vi "Write Topic Filter.vi"(8 "error in (no error)":errorcluster, 10 "Topic Filter":string, 11 "Subscription in":refnum<class "Subscription.lvclass">) -> (0 "error out":errorcluster, 3 "Subscription out":refnum<class "Subscription.lvclass">)   [LabVIEW 2013, in "MQTT Server.lvlib" / "Subscription.lvclass"]
uses:
  Subscription.lvclass
  Subscription.lvclass/Subscription.ctl
  TopicFilter/TopicFilter.lvclass/TopicFilter.ctl
  TopicFilter/TopicFilter.lvclass
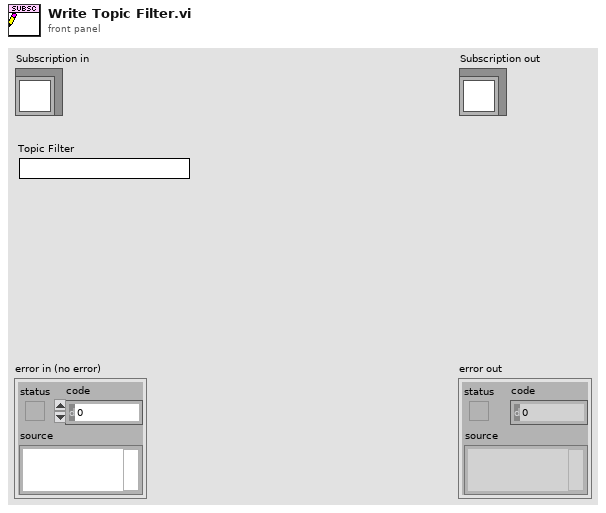
[diagram p1: front panel]
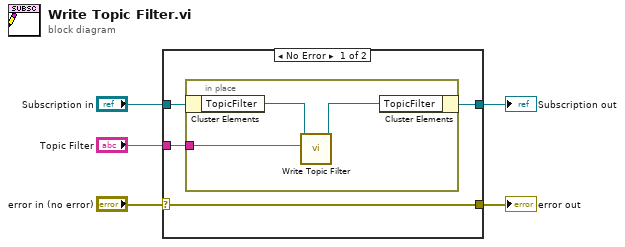
[diagram p0: block diagram]
diagram:
  n1 = case shown="No Error" "error in (no error)" {
    selector: "error in (no error)" -> [w9 w13]
    tunnel: [w9 w13] -> w4
    tunnel: [w6 w14] -> w2
    tunnel: "Subscription in" -> [w7 w14]
    tunnel: "Topic Filter" -> [w8 _]
    frame No Error {
      n2 = in-place {
        in-place-border: w8 -> [w12]
        n3 = in-place-cluster #1(w7) -> ("TopicFilter"=w11:refnum<class "TopicFilter.lvclass">)
        n4 = call "Write Topic Filter.vi"("Topic Filter"=w12, "TopicFilter in"=w11) -> ("TopicFilter out"=w10:refnum<class "TopicFilter.lvclass">)  [unwired: 9 in]
        n5 = in-place-cluster #1("TopicFilter"=w10) -> (w6:refnum<class "Subscription.lvclass">)
      }
    }
    frame Error {
    }
  }
  "error out" <- w4
  "Subscription out" <- w2
